vi "on-off.vi"() -> ()   [LabVIEW 2018]
panel:
  out "Slide":u8(slide) scale=0.0..100.0
  out "cooler":bool
  out "heater":bool
  in  "Dead Point":dbl
  in  "Setpoint":dbl
  out "Temperature":dbl
  in  "Input":dbl(knob) scale=0.0..100.0
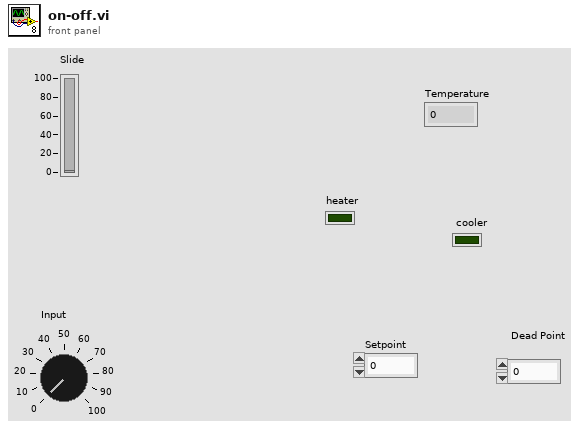
[diagram p1: front panel]
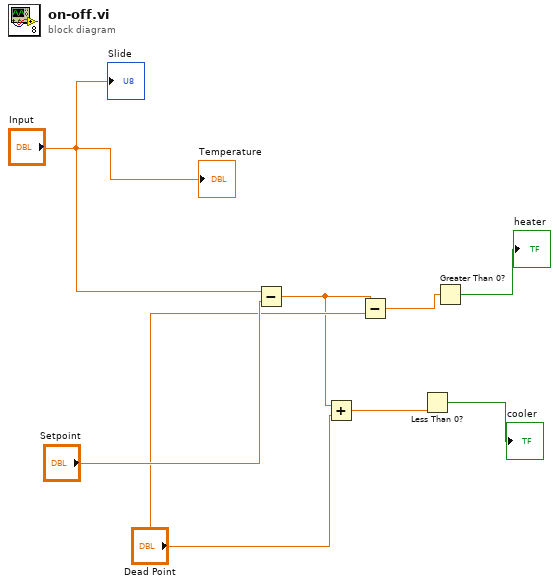
[diagram p0: block diagram]
diagram:
  n1 = Subtract(x="Input", y="Setpoint") -> (x-y=w1:dbl)
  n2 = Add(x=w1, y="Dead Point") -> (x+y=w8:dbl)
  n3 = Subtract(x=w1, y="Dead Point") -> (x-y=w5:dbl)
  n4 = Less Than 0?(x=w8) -> (x < 0?=→"cooler":bool)
  n5 = Greater Than 0?(x=w5) -> (x > 0?=→"heater":bool)
  "Temperature" <- "Input"
  "Slide" <- "Input"
